vi "Write.vi"(0 "System Interface":refnum<class "System Interface.lvclass">, 1 "Terminal":string="Output", 5 "Process Data":T1, 11 "Error In":errorcluster) -> (4 "System Interface out":refnum<class "System Interface.lvclass">, 15 "Error Out":errorcluster)   [LabVIEW 2020, in "Waveform(DBL) Array.lvlib"]
uses:
  <vilib>/ADAS Record/CustomDataTypes/Waveform(DBL) Array/Waveform(DBL) Array.lvlib
  <vilib>/FlexLogger/SDK/PluginSDK.lvlibp/PEFClasses/SDK/System Interface/System Interface.lvclass
  <vilib>/ADAS Record/CustomDataTypes/Waveform(DBL) Array/Process Data.ctl
  414300ae-2f3d-445e-aeca-488e23f625b8.vi
  414300ae-2f3d-445e-aeca-488e23f625b8.vi/fdfa6978-bdfc-4398-bc97-a01327bc44ce.vi
  414300ae-2f3d-445e-aeca-488e23f625b8.vi/409c1e6a-7c9d-40e3-aeb2-a56b28beb7cd.vi
  <vilib>/Utility/error.llb/Clear Errors.vi
  414300ae-2f3d-445e-aeca-488e23f625b8.vi/fdfa6978-bdfc-4398-bc97-a01327bc44ce.vi/cfd3d889-df14-41e5-9604-6a692e7e357a.vi
  414300ae-2f3d-445e-aeca-488e23f625b8.vi/409c1e6a-7c9d-40e3-aeb2-a56b28beb7cd.vi/55125485-cdad-4f1d-89b9-9bdf3801ca7d.vi
  414300ae-2f3d-445e-aeca-488e23f625b8.vi/409c1e6a-7c9d-40e3-aeb2-a56b28beb7cd.vi/c67d7082-f268-4082-9be0-83b0132da06c.vi
  414300ae-2f3d-445e-aeca-488e23f625b8.vi/409c1e6a-7c9d-40e3-aeb2-a56b28beb7cd.vi/1adf875c-fde0-460e-a784-90d221d44610.vi
  414300ae-2f3d-445e-aeca-488e23f625b8.vi/409c1e6a-7c9d-40e3-aeb2-a56b28beb7cd.vi/ef5cfb74-7e3c-4ca5-99ab-4d3670a506f3.vi
  <vilib>/FlexLogger/TestSystemInterface/Test System Interface.lvclass
  C:/Program Files/National Instruments/LabVIEW 2020/vi.lib/FlexLogger/SDK/PluginSDK.lvlibp/PEFClasses/SDK/System Interface/System Interface.lvclass
  <vilib>/ADAS Record/pefCommon/Tracing/SendGenericEvent.vi
  <vilib>/ADAS Record/CustomData/_Custom_RegisterType.vi
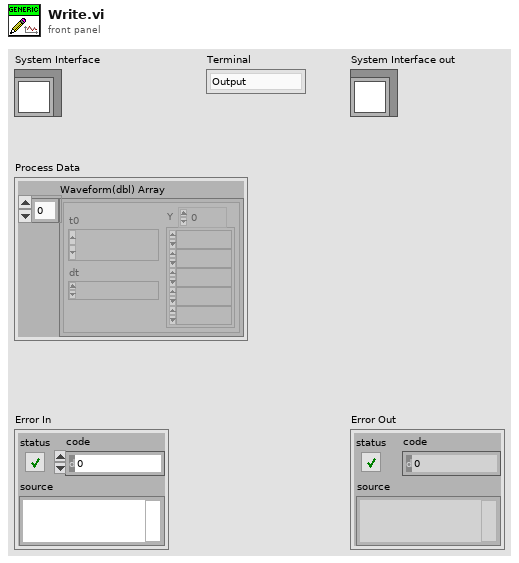
[diagram p1: front panel]
types:
  T1 = typedef "Waveform(DBL) Array.lvlib/Process Data.ctl" = cluster{"Waveform(dbl) Array":waveform(dbl)[]}
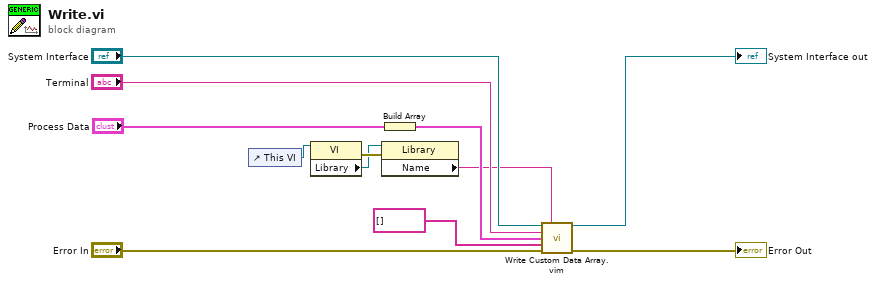
[diagram p0: block diagram]
diagram:
  n1 = control-ref of="This VI"() -> (w5:refnum<vi>)
  n2 = property class="VI"(reference=w5) -> (error out=w4:errorcluster, "Library"=w3:refnum<vi>)  [unwired: 1 in, 1 out]
  n3 = property class="Library"(reference=w3, error in=w4) -> ("Name"=w2:string)  [unwired: 2 out]
  n4 = Build Array("Process Data") -> (w7:T1[])
  n5 = call "Write Custom Data Array.vim"("System Interface"="System Interface", "Type"=w2, "Terminal"="Terminal", "Data"=w7, "Metadata"=string[] [], "error in (no error)"="Error In") -> ("System Interface out"=→"System Interface out":refnum<class "System Interface.lvclass">, "error out"=→"Error Out":errorcluster)  [unwired: 8 in]
